vi "TimeTracker.vi"(11 "Numeric in":i32=-1) -> (2 "Numeric out":i32, 3 "millisecond timer value":u32)   [LabVIEW 2018]
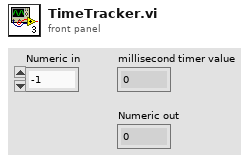
[diagram p1: front panel]
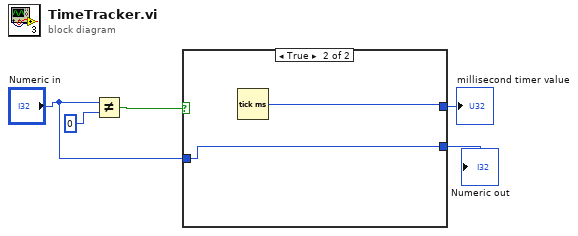
[diagram p0: block diagram]
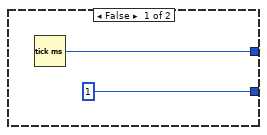
[diagram p2: hidden frame]
diagram:
  n1 = Not Equal?(x="Numeric in", y=0) -> (x != y?=w2:bool)
  n2 = case shown="True" w2 {
    tunnel: [w7 w8] -> w4
    tunnel: [1 w9] -> w5
    tunnel: "Numeric in" -> [_ w9]
    frame False {
      n3 = Tick Count (ms)() -> (millisecond timer value=w7:u32)
    }
    frame True {
      n4 = Tick Count (ms)() -> (millisecond timer value=w8:u32)
    }
  }
  "millisecond timer value" <- w4
  "Numeric out" <- w5
